vi "Create Bitfile Dependency.vi"(8 "error in (no error)":errorcluster, 10 "Bitfile Path":path, 11 "Item Ref in":T1 format="%.0x") -> (0 "error out":errorcluster, 3 "Device Ref out":T1 format="%.0x")   [LabVIEW 2015, in "Diagnostics Addon System Explorer.lvlib"]
uses:
  Diagnostics Addon System Explorer.lvlib
  <vilib>/NI Veristand/Custom Device API/Custom Device Item Ref.ctl
  Shared/SubVIs/GUID Lookup.vi
  <vilib>/Utility/MD5Checksum.llb/MD5Checksum File.vi
  <vilib>/NI Veristand/Custom Device API/NI VeriStand - Set Item Property.vi
  <vilib>/NI Veristand/Custom Device API/Set Item Property (Dependent File).vi
  <vilib>/NI Veristand/Custom Device API/NI VeriStand - Remove Item Property.vi
  Shared/Diagnostics Addon Shared.lvlib
  <vilib>/NI Veristand/Custom Device API/Custom Device API.lvlib
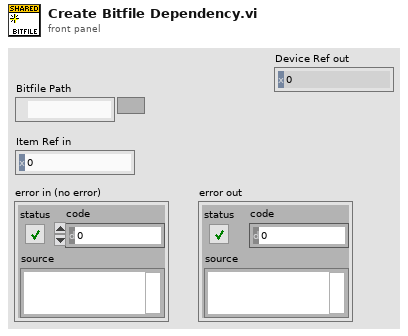
[diagram p1: front panel]
types:
  T1 = typedef "Custom Device API.lvlib/Custom Device Item Ref.ctl" = u64
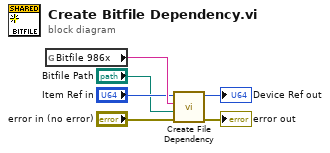
[diagram p0: block diagram]
diagram:
  n1 = global read "GUID Lookup.vi" "Bitfile 986x"() -> (w6:string)
  n2 = call "Create File Dependency.vi"("error in (no error)"="error in (no error)", "DLL Path"="Bitfile Path", "DLL Property Name"=w6, "Item Ref in"="Item Ref in") -> ("error out"=→"error out":errorcluster, "Item Ref out"=→"Device Ref out":T1)  [unwired: 6 in]
